vi "Stop Core.vi"(10 "final error code":i32, 11 "CS++GUIActor in":refnum<class "CS++GUIActor.lvclass">) -> (3 "CS++GUIActor out":refnum<class "CS++GUIActor.lvclass">)   [LabVIEW 2015, in "CS++GUIActor.lvlib" / "CS++GUIActor.lvclass"]
doc: "(<B>Filename</B>: Actor Framework.lvlib:Actor.lvclass:Stop Core.vi)\n\nDefines what the actor does before it stops. Use the <B>final error code</B> input to determine whether the actor shut down in response to an error.\n\nBy default, this method does nothing. A descendant class may override it to define behavior, such as shutting down any processes the actor initiated in its override of the Actor Core method."
uses:
  CS++GUIActor.lvclass
  CS++GUIActor.lvclass/CS++GUIActor.ctl
  CS++BaseActor/CS++BaseActor.lvclass
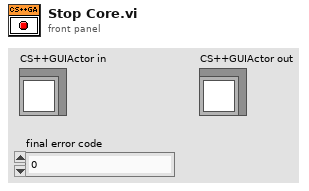
[diagram p1: front panel]
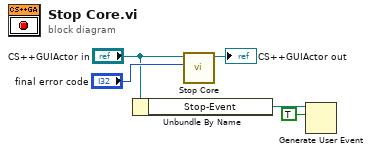
[diagram p0: block diagram]
diagram:
  n1 = Unbundle By Name("CS++GUIActor in") -> ("Stop-Event"=w2:refnum<user-event>)
  n2 = call-parent "Stop Core.vi"("final error code"="final error code", "CS++BaseActor in"="CS++GUIActor in") -> ("CS++BaseActor out"=→"CS++GUIActor out":refnum<class "CS++GUIActor.lvclass">)  [unwired: 9 in]
  n3 = Generate User Event(user event=w2, event data cluster=TRUE ("event data")) -> ()  [unwired: 2 in, 2 out]
